vi "Update Setpoint.vi"(8 "error in (no error)":errorcluster, 11 "MFC in":refnum<class "MFC.lvclass">) -> (0 "error out":errorcluster, 3 "MFC out":refnum<class "MFC.lvclass">)   [LabVIEW 2013, in "MFC.LVLIB" / "MFC.lvclass"]
uses:
  MFC.lvclass
  MFC.lvclass/MFC.ctl
  Read Setpoint.vi
  PluginInterface/PluginInterface.lvlibp/PluginInterfaceClass/Read DVR.vi
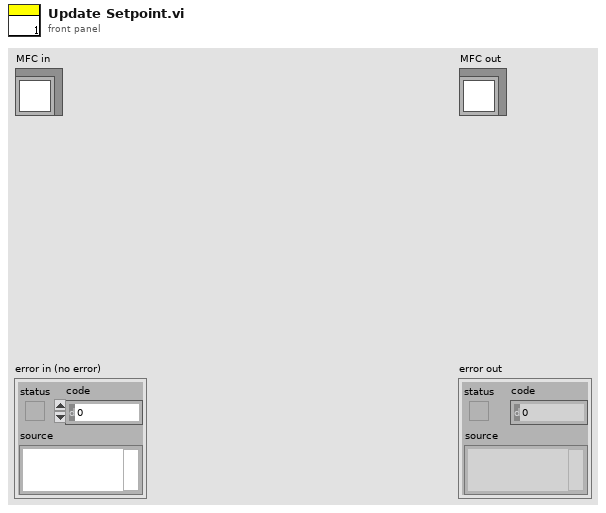
[diagram p1: front panel]
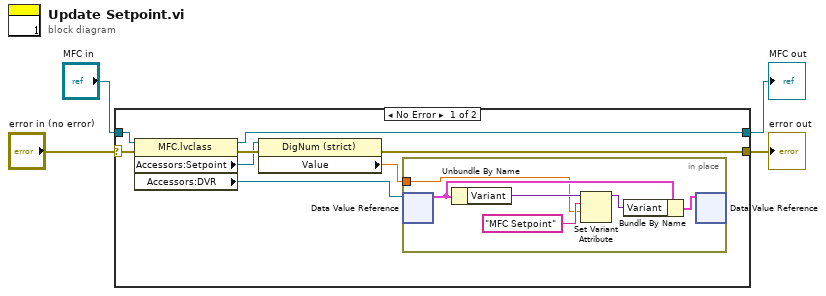
[diagram p0: block diagram]
diagram:
  n1 = case shown="No Error" "error in (no error)" {
    selector: "error in (no error)" -> [w8 w20]
    tunnel: [w5 w20] -> w1
    tunnel: [w11 w19] -> w2
    tunnel: "MFC in" -> [w7 w19]
    frame No Error {
      n2 = property class="MFC.lvclass"(reference=w7, error in=w8) -> (reference out=w11:refnum<class "MFC.lvclass">, error out=w12:errorcluster, "Accessors:Setpoint"=w9:refnum<vi>, "Accessors:DVR"=w10:refnum<data-value>)
      n3 = property class="DigNum (strict)"(reference=w9, error in=w12) -> (error out=w5:errorcluster, "Value"=w6:dbl)  [unwired: 1 out]
      n4 = in-place {
        in-place-border: w6 -> [w13]
        n5 = in-place-dvr #1(w10) -> (w15:cluster{"Array":string[], "Variant":variant})  [unwired: 1 out]
        n6 = Unbundle By Name(w15) -> ("Variant"=w17:variant)
        n7 = Set Variant Attribute(Variant=w17, name="MFC Setpoint", value=w13) -> (Variant out=w16:variant)  [unwired: 1 in, 2 out]
        n8 = Bundle By Name(cluster=w15, "Variant"=w16) -> (w18:cluster{"Array":string[], "Variant":variant})
        n9 = in-place-dvr #1(w18) -> ()  [unwired: 2 out]
      }
    }
    frame Error {
    }
  }
  "error out" <- w1
  "MFC out" <- w2
